vi "ArmLogic.vi"(7 "SensorError":bool, 8 "FuelArmSwitch":bool, 9 "PreviousFuelArm":bool, 10 "ArmSwitch":bool, 11 "PreviousArm":bool) -> (0 "FuelArm":bool, 3 "Arm":bool)   [LabVIEW 2016]
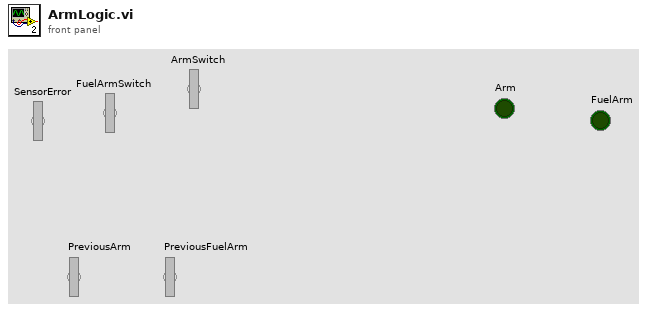
[diagram p1: front panel]
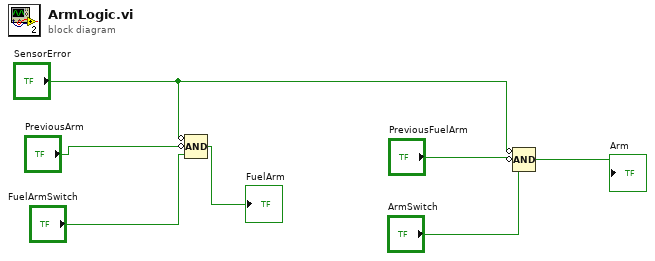
[diagram p0: block diagram]
diagram:
  n1 = Compound Arithmetic op=AND(invert "SensorError", invert "PreviousArm", "FuelArmSwitch") -> (→"FuelArm":bool)
  n2 = Compound Arithmetic op=AND(invert "SensorError", invert "PreviousFuelArm", "ArmSwitch") -> (→"Arm":bool)
